vi "Wait for Data.vi"(8 "error in (no error)":errorcluster, 10 "Initialize Time":bool, 11 "Pseudo PDC ID":i32) -> (0 "error out":errorcluster, 1 "PMU Status":T1(array[cluster]), 2 "PMU Data":T2(array[cluster]), 3 "Time Stamp":timestamp, 4 "Relative System Clock (ms)":dbl, 5 "Data OK":bool, 6 "dt (ms)":dbl)   [LabVIEW 2013, in "PMU Recorder Light.lvlib" / "Statnett C37.118 DLL.lvclass"]
uses:
  Statnett C37.118 DLL.lvclass
  c37118-dll/C37118-DLL.lvlib
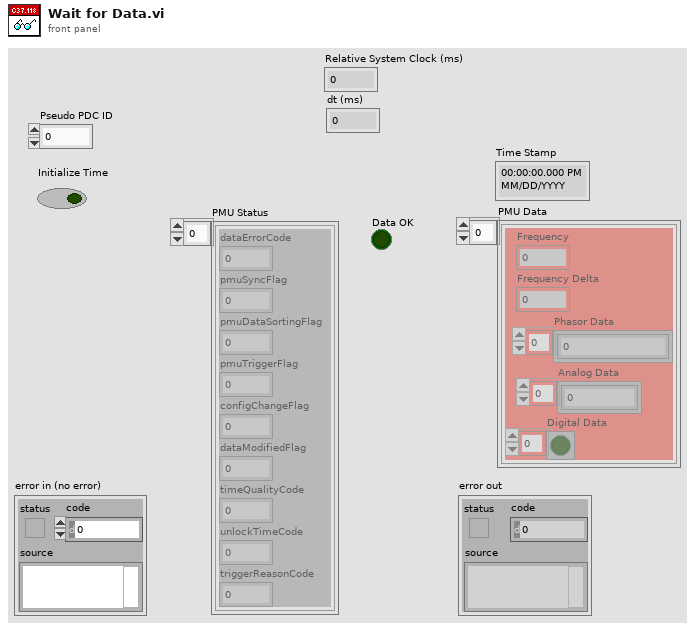
[diagram p1: front panel]
types:
  T1 = cluster{"dataErrorCode":u8, "pmuSyncFlag":u8, "pmuDataSortingFlag":u8, "pmuTriggerFlag":u8, "configChangeFlag":u8, "dataModifiedFlag":u8, "timeQualityCode":u8, "unlockTimeCode":u8, "triggerReasonCode":u8}[]
  T2 = cluster{"Frequency":sgl, "Frequency Delta":sgl, "Phasor Data":csg[], "Analog Data":sgl[], "Digital Data":bool[]}[]
  T3 = cluster{"Frequency":sgl, "Frequency Delta":sgl, "Phasor Data":csg[], "Analog Data":sgl[], "Digital Data":bool[]}
  T4 = cluster{"dataErrorCode":u8, "pmuSyncFlag":u8, "pmuDataSortingFlag":u8, "pmuTriggerFlag":u8, "configChangeFlag":u8, "dataModifiedFlag":u8, "timeQualityCode":u8, "unlockTimeCode":u8, "triggerReasonCode":u8}
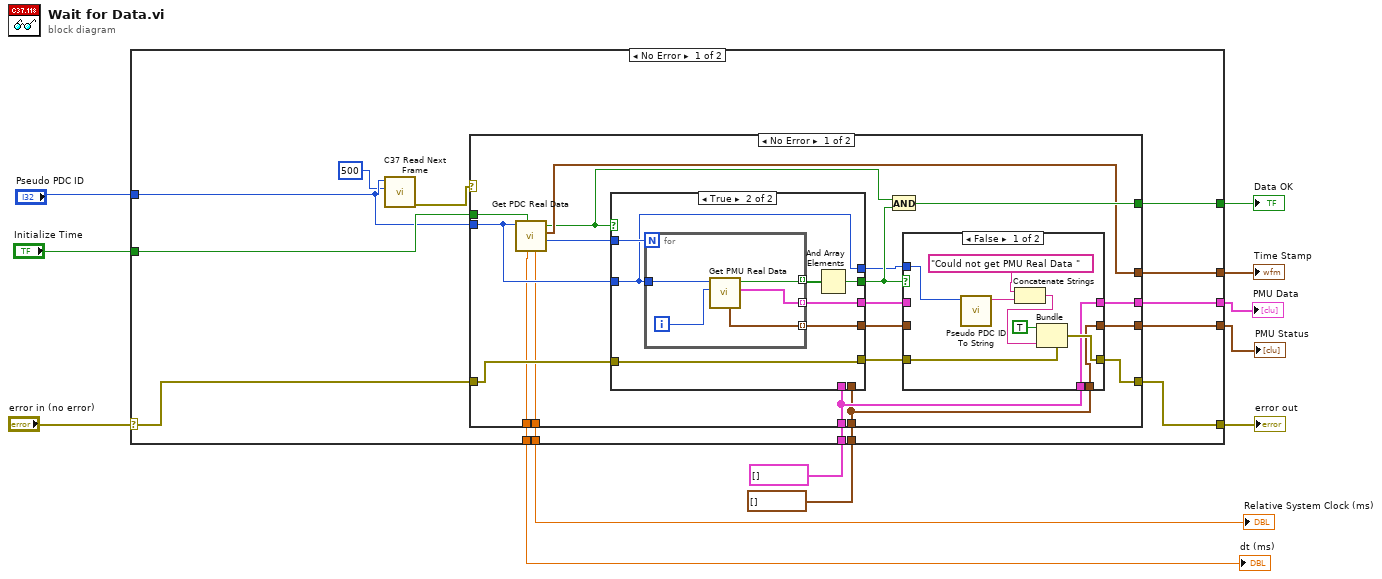
[diagram p0: block diagram]
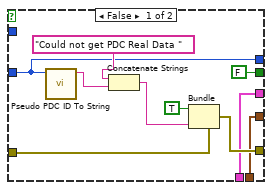
[diagram p3: hidden frame]
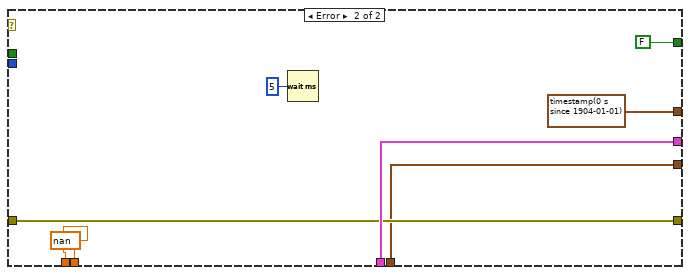
[diagram p4: hidden frame]
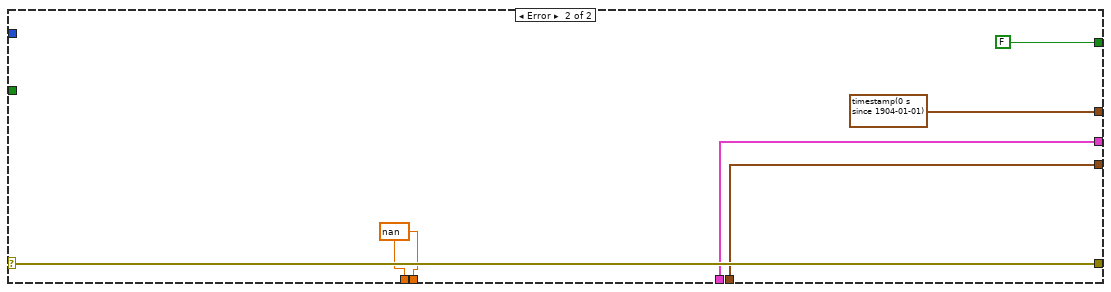
[diagram p5: hidden frame]
diagram:
  n1 = case shown="No Error" "error in (no error)" {
    selector: "error in (no error)" -> [w23 w92]
    tunnel: [w21 w92] -> w11
    tunnel: [w26 FALSE] -> w10
    tunnel: [w25 timestamp(0 s since 1904-01-01) ("Time Stamp")] -> w9
    tunnel: [w24 w87] -> w8
    tunnel: T2 [] -> [w22 w87]
    tunnel: "Pseudo PDC ID" -> [w17 _]
    tunnel: [w20 w89] -> w5
    tunnel: [w19 w89] -> w4
    tunnel: "Initialize Time" -> [w18 _]
    tunnel: [w14 w88] -> w2
    tunnel: T1 [] ("PMU Status") -> [w13 w88]
    frame No Error {
      n2 = call "C37 Read Next Frame.vi"("Timeout [ms]"=500 ("timeoutMs"), "Pseudo PDC ID"=w17) -> ("error out"=w15:errorcluster)  [unwired: 9 in]
      n3 = case shown="No Error" w15 {
        tunnel: w17 -> [w44 _]
        tunnel: [w43 FALSE] -> w26
        tunnel: [w42 timestamp(0 s since 1904-01-01) ("Time Stamp")] -> w25
        tunnel: [w35 w84] -> w24
        tunnel: w23 -> [w40 w83]
        tunnel: w22 -> [w33 w84]
        tunnel: [w36 w83] -> w21
        tunnel: [w32 w82] -> w20
        tunnel: [w31 w82] -> w19
        tunnel: w18 -> [w30 _]
        tunnel: [w28 w80] -> w14
        tunnel: w13 -> [w27 w80]
        frame No Error {
          n4 = call "Get PDC Real Data.vi"("Initialize Time"=w30, "Pseudo PDC ID"=w44) -> ("Number of PMUs"=w45:i32, "Time Stamp"=w42:timestamp, "Data OK"=w41:bool, "Relative System Clock (ms)"=w32:dbl, "dt (ms)"=w31:dbl)  [unwired: 4 in, 1 out]
          n5 = case shown="True" w41 {
            tunnel: w45 -> [_ w74]
            tunnel: w44 -> [w60 w69]
            tunnel: [FALSE w72] -> w39
            tunnel: [w59 w71] -> w38
            tunnel: w40 -> [w64 w70]
            tunnel: [w62 w70] -> w37
            tunnel: w33 -> [w59 _]
            tunnel: [w60 w69] -> w34
            tunnel: [w58 w68] -> w29
            tunnel: w27 -> [w58 _]
            frame False {
              n6 = call "Pseudo PDC ID To String.vi"("Pseudo PDC ID"=w60) -> ("String"=w66:string)  [unwired: 10 in]
              n7 = Concatenate Strings("Could not get PDC Real Data " ("source"), w66) -> (w63:string)
              n8 = Bundle(cluster=w64, "status"=TRUE, "source"=w63) -> (w62:errorcluster)  [unwired: 1 in]
            }
            frame True {
              n9 = for {
                N: w74 -> [_]
                tunnel: w69 -> [w78]
                tunnel: [w77] -> w73 mode=indexing
                tunnel: [w76] -> w71 mode=indexing
                tunnel: [w75] -> w68 mode=indexing
                i -> [w79]
                n10 = call "Get PMU Real Data.vi"("PMU Index"=w79, "Pseudo PDC ID"=w78) -> ("PMU Data"=w76:T3, "Data OK"=w77:bool, "status"=w75:T4)  [unwired: 7 in]
              }
              n11 = And Array Elements(Boolean array=w73) -> (logical AND=w72:bool)
            }
          }
          n12 = And(x=w41, y=w39) -> (x .and. y?=w43:bool)
          n13 = case shown="False" w39 {
            tunnel: w38 -> [_ w56]
            tunnel: w37 -> [w50 w57]
            tunnel: [w49 w57] -> w36
            tunnel: [w47 w56] -> w35
            tunnel: w34 -> [w54 _]
            tunnel: w33 -> [w47 _]
            tunnel: w29 -> [_ w55]
            tunnel: [w46 w55] -> w28
            tunnel: w27 -> [w46 _]
            frame False {
              n14 = call "Pseudo PDC ID To String.vi"("Pseudo PDC ID"=w54) -> ("String"=w53:string)  [unwired: 10 in]
              n15 = Concatenate Strings("Could not get PMU Real Data " ("source"), w53) -> (w48:string)
              n16 = Bundle(cluster=w50, "status"=TRUE, "source"=w48) -> (w49:errorcluster)  [unwired: 1 in]
            }
            frame True {
            }
          }
        }
        frame Error {
          w82 = nan ("Relative System Clock (ms)")
          n17 = Wait (ms)(milliseconds to wait=u32 5) -> ()  [unwired: 1 out]
        }
      }
    }
    frame Error {
      w89 = nan ("dt (ms)")
    }
  }
  "error out" <- w11
  "Data OK" <- w10
  "Time Stamp" <- w9
  "PMU Data" <- w8
  "Relative System Clock (ms)" <- w5
  "dt (ms)" <- w4
  "PMU Status" <- w2
